vi "Read Column Headers.vi"(8 "error in (no error)":errorcluster, 11 "FastTreeView in":refnum<class "FastTreeView.lvclass">) -> (0 "error out":errorcluster, 2 "Column Headers":string[](array[string]), 3 "FastTreeView out":refnum<class "FastTreeView.lvclass">)   [LabVIEW 2025, in "FastTreeView.lvclass"]
uses:
  FastTreeView.lvclass
  FastTreeView.lvclass/FastTreeView.ctl
  C:/Git/FastTreeView/FastTreeView/LV/FastTreeView/dll/FastTreeView.dll
  dll/FastTreeView.dll
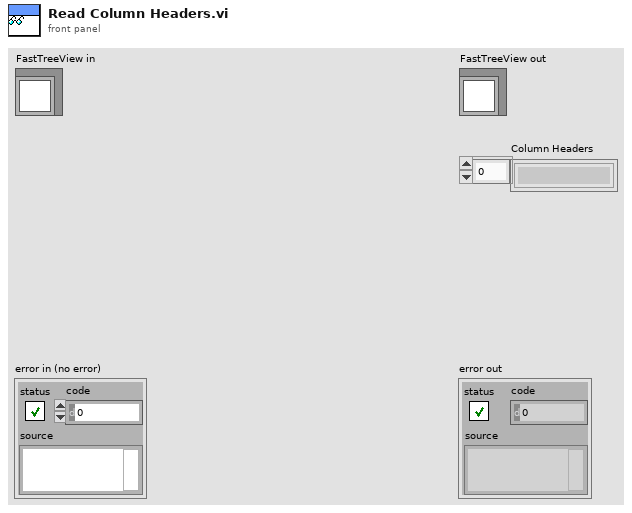
[diagram p1: front panel]
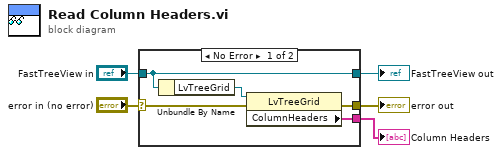
[diagram p0: block diagram]
diagram:
  n1 = case shown="No Error" "error in (no error)" {
    selector: "error in (no error)" -> [w7 w11]
    tunnel: [w6 w11] -> w4
    tunnel: [w10 w12] -> w2
    tunnel: "FastTreeView in" -> [w10 w12]
    tunnel: [w8 _] -> w1
    frame No Error {
      n2 = Unbundle By Name(w10) -> ("LvTreeGrid"=w9:refnum<k24>)
      n3 = property class="LvTreeGrid"(reference=w9, error in=w7) -> (error out=w6:errorcluster, "ColumnHeaders"=w8:string[])  [unwired: 1 out]
    }
    frame Error {
    }
  }
  "error out" <- w4
  "FastTreeView out" <- w2
  "Column Headers" <- w1
